vi "configure.vi"(8 "error in (no error)":errorcluster, 11 "GenericPlugin in":refnum<class "FPGAWrapperMH120124FrameScan_PXI7813R.lvclass">) -> (0 "error out":errorcluster, 3 "GenericPlugin out":refnum<class "FPGAWrapperMH120124FrameScan_PXI7813R.lvclass">)   [LabVIEW 2010, in "FPGAWrapperMH120124FrameScan_PXI7813R.lvclass"]
doc: "The dynamic dispatch version of this VI loads and displays the configuration file associated with the plug-in object. The user modify and save the configuration data."
uses:
  FPGAWrapperMH120124FrameScan_PXI7813R.lvclass
  fpgaVIsAndControls/inverse_enum.ctl
  fpgaVIsAndControls/DDS_board_init_cluster.ctl
  FPGAWrapperMH120124FrameScan_PXI7813R.lvclass/FPGAWrapperMH120124FrameScan_PXI7813R.ctl
  common/classes/GenericComponent/GenericComponent/GenericComponent.lvclass
panel:
  in  "Tab Control":T1(tab)
  in  "integration delay (iterations)":u32
  in  "integration delay (pixels)":u32
  in  "OSK select":bool=TRUE
  in  "AOD center frequ. (Hz)":dbl[unit]=94000000.0
  in  "AOD Bandwidth":dbl[unit]=34000000.0
  in  "inverse?":T2
  in  "AOD amplitude":u16=3400
  in  "AOD equilibration time":dbl[unit]=9.999999999999999e-06
  in  "DDS board initialization parameters":T3={"Bypass PLL"=FALSE, "PLL Range"=TRUE, "Update Clock"=FALSE, "Triangle "=FALSE, "SDO Active"=FALSE, "LSB First"=FALSE, "OSK Int"=FALSE, "Output Shaped Keying Enable"=TRUE, "Bypass Sinc"=FALSE, "Digital Part"=TRUE, "OutPut DAC"=TRUE, "Control DAC"=FALSE, "Comparator"=FALSE, "Modus"=0, "Multiplier Value"=15} {"Modus" scale=0.0..4.0}
  in  "cancel":bool
  in  "save":bool
  out "Configuration name":string
  # "Configure FPGAWrapperFrameScan"
  # "The TrajectoryMG100122AODFrameScan component controls the frame scan trajectory for the FPGA.\n\nEach FPGA controls the home built direct digital synthesizer (DDS) board that synthesizes the wave forms for the acousto-optic deflectors (AOD)."
  # "Settings for the direct digital synthesizer and acousto-optic de-flectors. See wiki page and manuals for standard values."
  # "FSK"
  # "Ramped"
  # "FSK"
  # "Chirp Modus"
  # "Unramped"
  # "BPSK"
  # "Single Tone"
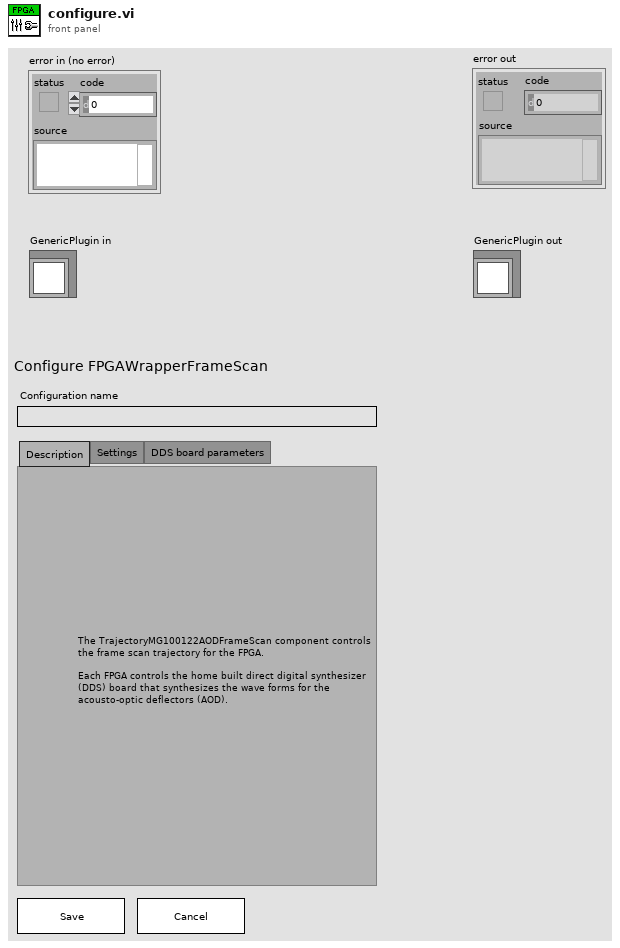
[diagram p1: front panel]
types:
  T1 = enum32{"Description", "Settings", "DDS board parameters"}
  T2 = typedef "inverse_enum.ctl" = enum16{"normal", "x inversed", "y inversed", "x & y inversed"}
  T3 = typedef "DDS_board_init_cluster.ctl" = cluster{"Bypass PLL":bool, "PLL Range":bool, "Update Clock":bool, "Triangle ":bool, "SDO Active":bool, "LSB First":bool, "OSK Int":bool, "Output Shaped Keying Enable":bool, "Bypass Sinc":bool, "Digital Part":bool, "OutPut DAC":bool, "Control DAC":bool, "Comparator":bool, "Modus":u8, "Multiplier Value":u8}
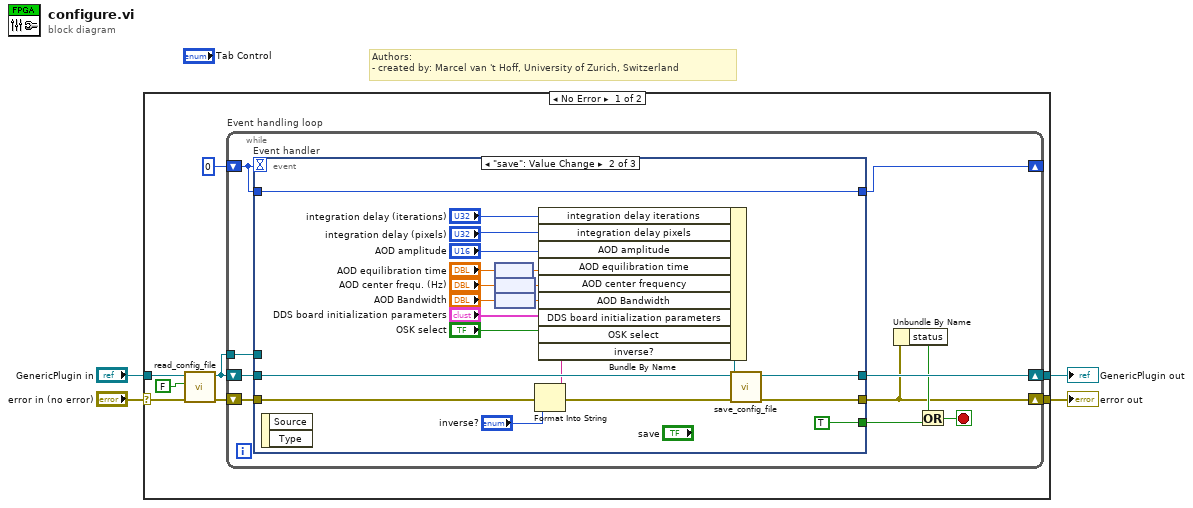
[diagram p0: block diagram]
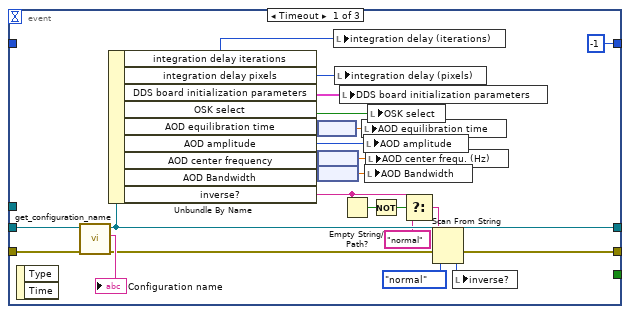
[diagram p2: hidden frame]
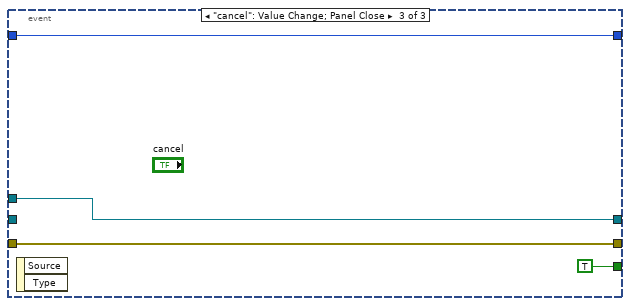
[diagram p3: hidden frame]
diagram:
  # "Authors: \n- created by: Marcel van 't Hoff, University of Zurich, Switzerland"
  n1 = case shown="No Error" "error in (no error)" {
    selector: "error in (no error)" -> [w9 w74]
    tunnel: [w11 w74] -> w2
    tunnel: [w10 w73] -> w1
    tunnel: "GenericPlugin in" -> [w7 w73]
    frame No Error {
      n2 = call-dynamic "read_config_file.vi"("error in (no error)"=w9, "force load?"=FALSE, "GenericPlugin in"=w7) -> ("error out"=w8:errorcluster, "GenericPlugin out"=w5:refnum<class "FPGAWrapperMH120124FrameScan_PXI7813R.lvclass">)  [unwired: 7 out]
      n3 = while "Event handling loop" {
        shift-right: [w20] -> _
        shift-left: 0 -> [w21]
        shift-right: [w16] -> w11
        shift-left: w8 -> [w22]
        shift-right: [w18] -> w10
        shift-left: w5 -> [w19]
        tunnel: w5 -> [w13]
        stop <- w15 stop-if-true
        n4 = event "Event handler" shown="[1] \"save\": Value Change" {
          selector: _ -> [_ _ _]
          dyn-events: _ -> [_ _ _]
          timeout: w21 -> [_ _ _]
          tunnel: w22 -> [w46 w56 w71]
          tunnel: [-1 w68 w72] -> w20
          tunnel: w21 -> [_ w68 w72]
          tunnel: [w35 w67 w71] -> w16
          tunnel: [_ TRUE TRUE] -> w14
          tunnel: w19 -> [w45 w57 _]
          tunnel: [w43 w66 w69] -> w18
          tunnel: w13 -> [_ _ w69]
          event Timeout {
            n5 = event-data() -> ()  [unwired: 3 out]
            n6 = call "get_configuration_name.vi"("error in (no error)"=w46, "GenericPlugin.lvclass in"=w45) -> ("error out"=w36:errorcluster, "configuration name"=→"Configuration name":string, "GenericPlugin.lvclass out"=w43:refnum<class "FPGAWrapperMH120124FrameScan_PXI7813R.lvclass">)  [unwired: 7 in]
            n7 = Unbundle By Name(w43) -> ("integration delay iterations"=w23:u32, "integration delay pixels"=w24:u32, "DDS board initialization parameters"=w40:T3, "OSK select"=w41:bool, "AOD equilibration time"=w37:dbl, "AOD amplitude"=w42:u16, "AOD center frequency"=w38:dbl, "AOD Bandwidth"=w39:dbl, "inverse?"=w30:string)
            n8 = node(w37) -> (w27:dbl[unit])
            n9 = node(w38) -> (w26:dbl[unit])
            n10 = node(w39) -> (w25:dbl[unit])
            n11 = local write "integration delay (iterations)"(w23) -> ()
            n12 = local write "integration delay (pixels)"(w24) -> ()
            n13 = local write "DDS board initialization parameters"(w40) -> ()
            n14 = Empty String/Path?(string/path=w30) -> (empty?=w32:bool)
            n15 = local write "AOD equilibration time"(w27) -> ()
            n16 = local write "AOD amplitude"(w42) -> ()
            n17 = local write "AOD Bandwidth"(w25) -> ()
            n18 = local write "AOD center frequ. (Hz)"(w26) -> ()
            n19 = local write "OSK select"(w41) -> ()
            n20 = Not(x=w32) -> (.not. x?=w31:bool)
            n21 = Select(t=w30, s=w31, f="normal") -> (s? t:f=w29:string)
            n22 = Scan From String(input string=w29, error in=w36, default 1=inverse_enum."normal" ("inverse?")) -> (error out=w35:errorcluster, output 1=w33:T2)  [unwired: 2 in, 2 out]
            n23 = local write "inverse?"(w33) -> ()
          }
          event "save": Value Change {
            n24 = event-data() -> ()  [unwired: 3 out]
            n25 = node("AOD equilibration time") -> (w52:dbl)
            n26 = node("AOD center frequ. (Hz)") -> (w51:dbl)
            n27 = node("AOD Bandwidth") -> (w50:dbl)
            n28 = Format Into String(error in=w56, "inverse?") -> (resulting string=w53:string, error out=w55:errorcluster)  [unwired: 2 in]
            n29 = Bundle By Name(cluster=w57, "integration delay iterations"="integration delay (iterations)", "integration delay pixels"="integration delay (pixels)", "AOD amplitude"="AOD amplitude", "AOD equilibration time"=w52, "AOD center frequency"=w51, "AOD Bandwidth"=w50, "DDS board initialization parameters"="DDS board initialization parameters", "OSK select"="OSK select", "inverse?"=w53) -> (w62:refnum<class "FPGAWrapperMH120124FrameScan_PXI7813R.lvclass">)
            n30 = call-dynamic "save_config_file.vi"("error in (no error)"=w55, "GenericPlugin in"=w62) -> ("error out"=w67:errorcluster, "GenericPlugin out"=w66:refnum<class "FPGAWrapperMH120124FrameScan_PXI7813R.lvclass">)  [unwired: 2 in, 6 out]
          }
          event "cancel": Value Change; Panel Close {
            n31 = event-data() -> ()  [unwired: 3 out]
          }
        }
        n32 = Unbundle By Name(w16) -> ("status"=w17:bool)
        n33 = Or(x=w17, y=w14) -> (x .or. y?=w15:bool)
      }
    }
    frame Error {
    }
  }
  "error out" <- w2
  "GenericPlugin out" <- w1
